vi "Parse Response.vi"(8 "error in (no error)":errorcluster, 10 "Command":T1, 11 "ESM303 in":refnum<class "ESM303.lvclass">) -> (0 "error out":errorcluster, 3 "ESM303 out":refnum<class "ESM303.lvclass">)   [LabVIEW 2018, in "ESM303.lvlib" / "ESM303.lvclass"]
uses:
  ESM303.lvclass
  builds/Force Test Stand.lvlibp/Custom Controls/Commands.ctl
  ESM303.lvclass/ESM303.ctl
  builds/Force Test Stand.lvlibp/Custom Controls/Crosshead Status.ctl
  builds/Force Test Stand.lvlibp/Custom Controls/Operating Mode.ctl
  builds/Force Test Stand.lvlibp/Custom Controls/Limit Switch Status.ctl
  builds/Force Test Stand.lvlibp/Custom Controls/Travel Units.ctl
  builds/Force Test Stand.lvlibp/Custom Controls/Speed Units.ctl
  builds/Force Test Stand.lvlibp/Custom Controls/Force Units.ctl
  builds/Force Test Stand.lvlibp/Force Test Stand.lvclass
  C:/Users/Ron.Dexter.LUMINARTECH/Desktop/builds/Force Test Stand.lvlibp/Force Test Stand.lvclass
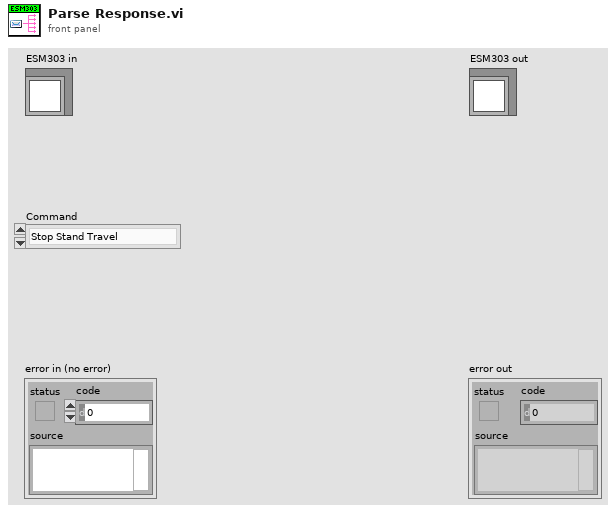
[diagram p1: front panel]
types:
  T1 = typedef "Force Test Stand.lvlibp/Force Test Stand.lvclass/Commands.ctl" = enum16{"Stop Stand Travel", "Start Travel Down (Left)", "Start Travel Up (Right)", "Get Travel Upper Limit", "Get Travel Lower Limit", "Set Travel Upper Limit", "Set Travel Lower Limit", "Get Travel Value", "Set Travel Units (mm)", "Set Travel Units (in)", "Reset Travel to Zero", "Get Speed ", "Set Speed", "Set Speed to Min", "Set Speed to Max", "Get Force Value", "Get Force Units", "Set Force Units (lbF)", "Get Stand Status", "Set Cycle Mode", "Set Limit Mode", "Set Manual Mode", "Set No. Cycles", "Get Travel/Force Values", "Get Completed Cycles", "Get Cycles Setpoint", "Reset Cycles Counter", "Zero Force Gauge", "Set Force Upper Limit", "Set Force Lower Limit", "Get Travel Units", "Get Speed Units", "Default", "Set Force Units (N)", "Set Force Units (kgF)", "Set Force Units (ozF)", "Set Force Units (gF)", "Set Force Real Time Mode", "Set Force Peak Tension Mode", "Set Force Peak Compression Mode", "Set Force High Set-Point", "Set Force Low Set-Point", "Gauge Transmit with Units", "Gauge Transmit w/o Units", "Get Peak Compression Force", "Get Peak Tension Force", "Get Real Time Force", "Disable Force High Limit", "Disable Force Low Limit", "Send Speed Setting to Stand"}
  T2 = typedef "Force Test Stand.lvlibp/Force Test Stand.lvclass/Limit Switch Status.ctl" = enum16{"At Upper Limit", "At Lower Limit", "At No Limit"}
  T3 = typedef "Force Test Stand.lvlibp/Force Test Stand.lvclass/Crosshead Status.ctl" = enum16{"Moving Up (Right)", "Moving Down (Left)", "Stopped"}
  T4 = typedef "Force Test Stand.lvlibp/Force Test Stand.lvclass/Operating Mode.ctl" = enum16{"Cycle", "Limit", "Manual"}
  T5 = typedef "Force Test Stand.lvlibp/Force Test Stand.lvclass/Travel Units.ctl" = enum16{"in", "mm"}
  T6 = typedef "Force Test Stand.lvlibp/Force Test Stand.lvclass/Speed Units.ctl" = enum16{"in/min", "mm/min"}
  T7 = typedef "Force Test Stand.lvlibp/Force Test Stand.lvclass/Force Units.ctl" = enum16{"lbF", "ozF", "gF", "kgF", "N", "kN", "mN"}
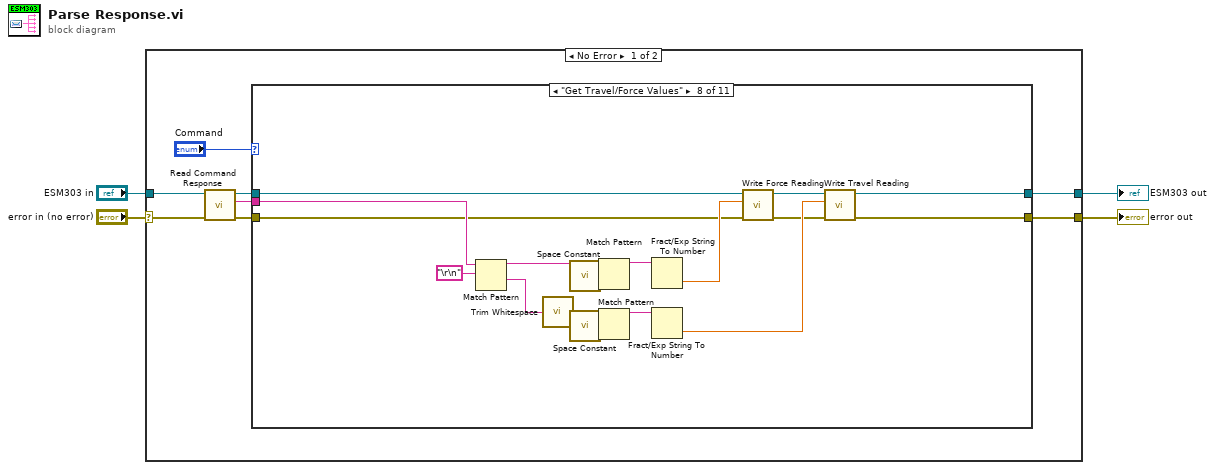
[diagram p0: block diagram]
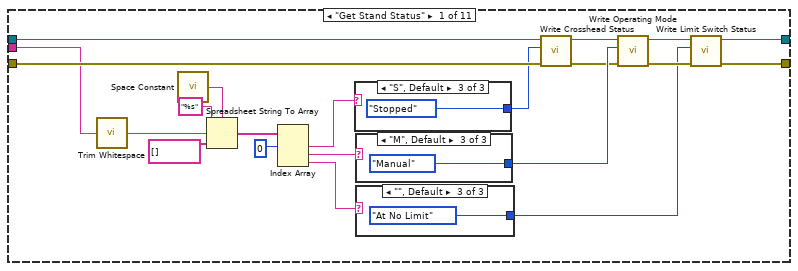
[diagram p2: hidden frame]
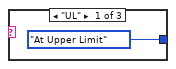
[diagram p3: hidden frame]
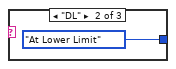
[diagram p4: hidden frame]
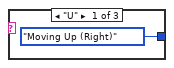
[diagram p5: hidden frame]
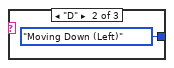
[diagram p6: hidden frame]
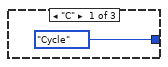
[diagram p7: hidden frame]
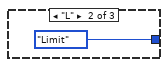
[diagram p8: hidden frame]
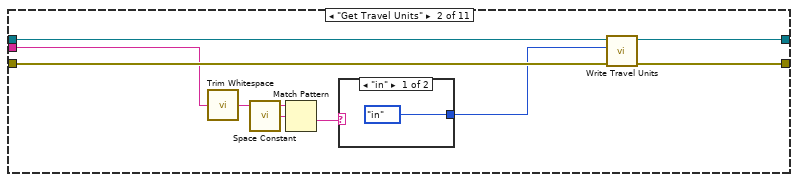
[diagram p9: hidden frame]
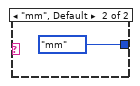
[diagram p10: hidden frame]
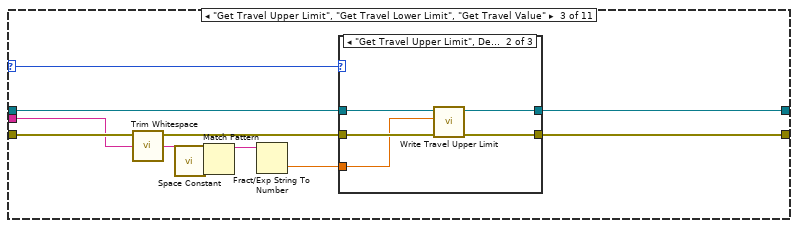
[diagram p11: hidden frame]
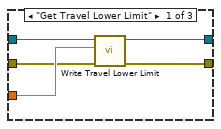
[diagram p12: hidden frame]
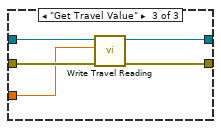
[diagram p13: hidden frame]
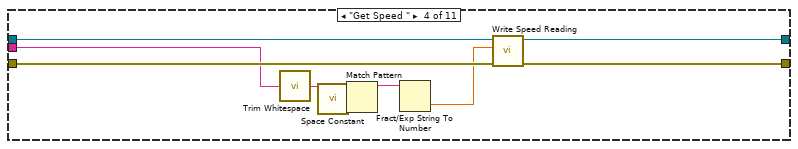
[diagram p14: hidden frame]
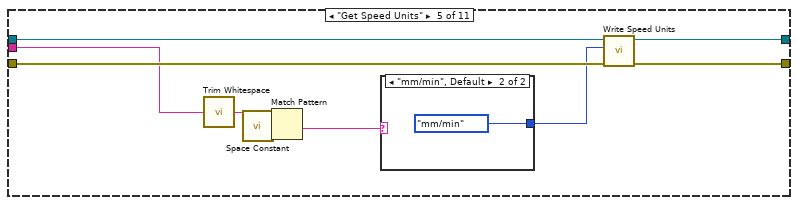
[diagram p15: hidden frame]
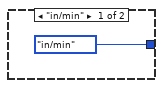
[diagram p16: hidden frame]
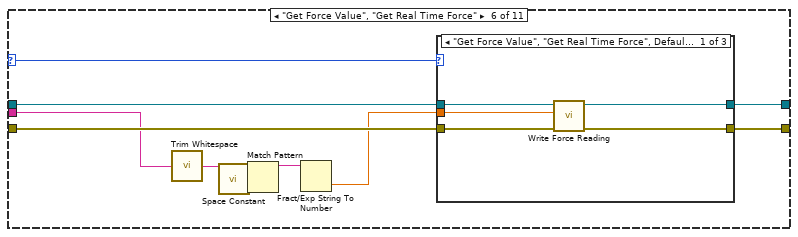
[diagram p17: hidden frame]
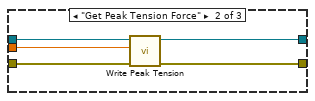
[diagram p18: hidden frame]
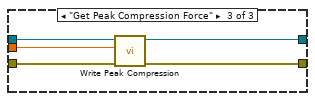
[diagram p19: hidden frame]
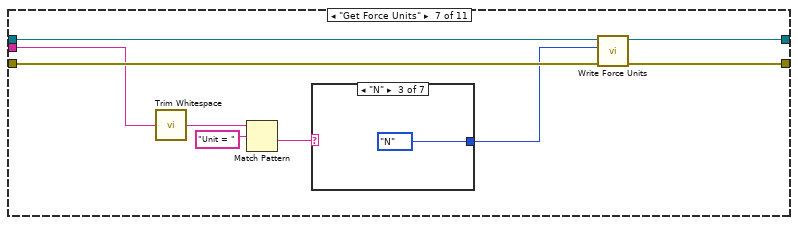
[diagram p20: hidden frame]
diagram:
  n1 = case shown="No Error" "error in (no error)" {
    selector: "error in (no error)" -> [w12 w176]
    tunnel: [w5 w176] -> w3
    tunnel: [w8 w175] -> w1
    tunnel: "ESM303 in" -> [w11 w175]
    frame No Error {
      n2 = call "Read Command Response.vi"("error in (no error)"=w12, "ESM303 in"=w11) -> ("error out"=w6:errorcluster, "Command Response"=w7:string, "ESM303 out"=w10:refnum<class "ESM303.lvclass">)  [unwired: 7 in]
      n3 = case shown="\"Get Travel/Force Values\"" "Command" {
        selector: "Command" -> [_ _ w63 _ _ w99 _ _ _ _ _]
        tunnel: w10 -> [w26 w49 w62 w83 w95 w108 w132 w149 w165 w171 w174]
        tunnel: [w18 w47 w57 w87 w94 w107 w130 w144 w163 w169 w174] -> w8
        tunnel: w7 -> [w14 w44 w55 w80 w89 w101 w125 w156 w160 w167 _]
        tunnel: w6 -> [w25 w48 w61 w82 w92 w106 w131 w146 w164 w170 w173]
        tunnel: [w17 w46 w56 w86 w93 w105 w129 w143 w162 w168 w173] -> w5
        frame "Get Stand Status" {
          n4 = call <vilib>:"Trim Whitespace.vi"("string"=w14) -> ("trimmed string"=w13:string)  [unwired: 1 in]
          n5 = call <vilib>:"Space Constant.vi"() -> ("String"=w15:string)
          n6 = Spreadsheet String To Array(delimiter (Tab)=w15, format string="%s", spreadsheet string=w13, array type (2D Dbl)=string[] []) -> (array=w31:string[])
          n7 = Index Array(array=w31, index #1=0) -> (element #1=w27:string, element #2=w29:string, element #3=w21:string)  [unwired: 2 in]
          n8 = case shown="\"S\", Default" w27 {
            tunnel: [Crosshead_Status."Moving Up (Right)" ("Crosshead Status") Crosshead_Status."Moving Down (Left)" ("Crosshead Status") Crosshead_Status."Stopped" ("Crosshead Status")] -> w22
            frame "U" {
            }
            frame "D" {
            }
            frame "S", Default {
            }
          }
          n9 = case shown="\"M\", Default" w29 {
            tunnel: [Operating_Mode."Cycle" ("Operating Mode") Operating_Mode."Limit" ("Operating Mode") Operating_Mode."Manual" ("Operating Mode")] -> w28
            frame "C" {
            }
            frame "L" {
            }
            frame "M", Default {
            }
          }
          n10 = case shown="\"\", Default" w21 {
            tunnel: [Limit_Switch_Status."At Upper Limit" ("Limit Switch Status") Limit_Switch_Status."At Lower Limit" ("Limit Switch Status") Limit_Switch_Status."At No Limit" ("Limit Switch Status")] -> w16
            frame "UL" {
            }
            frame "DL" {
            }
            frame "", Default {
            }
          }
          n11 = call "Write Crosshead Status.vi"("error in (no error)"=w25, "Crosshead Status"=w22, "Force Test Stand in"=w26) -> ("error out"=w23:errorcluster, "Force Test Stand out"=w24:refnum<class "ESM303.lvclass">)  [unwired: 7 in]
          n12 = call "Write Operating Mode.vi"("error in (no error)"=w23, "Operating Mode"=w28, "Force Test Stand in"=w24) -> ("error out"=w19:errorcluster, "Force Test Stand out"=w20:refnum<class "ESM303.lvclass">)  [unwired: 7 in]
          n13 = call "Write Limit Switch Status.vi"("error in (no error)"=w19, "Limit Switch Status"=w16, "Force Test Stand in"=w20) -> ("error out"=w17:errorcluster, "Force Test Stand out"=w18:refnum<class "ESM303.lvclass">)  [unwired: 7 in]
        }
        frame "Get Travel Units" {
          n14 = call <vilib>:"Trim Whitespace.vi"("string"=w44) -> ("trimmed string"=w43:string)  [unwired: 1 in]
          n15 = call <vilib>:"Space Constant.vi"() -> ("String"=w51:string)
          n16 = Match Pattern(string=w43, regular expression=w51) -> (after substring=w50:string)  [unwired: 1 in, 3 out]
          n17 = case shown="\"in\"" w50 {
            tunnel: [Travel_Units."in" ("Travel Units") Travel_Units."mm" ("Travel Units")] -> w45
            frame "in" {
            }
            frame "mm", Default {
            }
          }
          n18 = call "Write Travel Units.vi"("error in (no error)"=w48, "Travel Units"=w45, "Force Test Stand in"=w49) -> ("error out"=w46:errorcluster, "Force Test Stand out"=w47:refnum<class "ESM303.lvclass">)  [unwired: 7 in]
        }
        frame "Get Travel Upper Limit", "Get Travel Lower Limit", "Get Travel Value" {
          n19 = call <vilib>:"Trim Whitespace.vi"("string"=w55) -> ("trimmed string"=w54:string)  [unwired: 1 in]
          n20 = call <vilib>:"Space Constant.vi"() -> ("String"=w59:string)
          n21 = Match Pattern(string=w54, regular expression=w59) -> (before substring=w58:string)  [unwired: 1 in, 3 out]
          n22 = Fract/Exp String To Number(string=w58) -> (number=w60:dbl)  [unwired: 3 in, 1 out]
          n23 = case shown="\"Get Travel Upper Limit\", Default" w63 {
            tunnel: w62 -> [w68 w73 w76]
            tunnel: [w67 w72 w74] -> w57
            tunnel: w61 -> [w65 w71 w78]
            tunnel: [w64 w70 w77] -> w56
            tunnel: w60 -> [w66 w69 w75]
            frame "Get Travel Lower Limit" {
              n24 = call "Write Travel Lower Limit.vi"("error in (no error)"=w65, "Travel Lower Limit"=w66, "Force Test Stand in"=w68) -> ("error out"=w64:errorcluster, "Force Test Stand out"=w67:refnum<class "ESM303.lvclass">)  [unwired: 7 in]
            }
            frame "Get Travel Upper Limit", Default {
              n25 = call "Write Travel Upper Limit.vi"("error in (no error)"=w71, "Travel Upper Limit"=w69, "Force Test Stand in"=w73) -> ("error out"=w70:errorcluster, "Force Test Stand out"=w72:refnum<class "ESM303.lvclass">)  [unwired: 7 in]
            }
            frame "Get Travel Value" {
              n26 = call "Write Travel Reading.vi"("error in (no error)"=w78, "Travel Reading"=w75, "Force Test Stand in"=w76) -> ("error out"=w77:errorcluster, "Force Test Stand out"=w74:refnum<class "ESM303.lvclass">)  [unwired: 7 in]
            }
          }
        }
        frame "Get Speed " {
          n27 = call <vilib>:"Trim Whitespace.vi"("string"=w80) -> ("trimmed string"=w79:string)  [unwired: 1 in]
          n28 = call <vilib>:"Space Constant.vi"() -> ("String"=w85:string)
          n29 = Match Pattern(string=w79, regular expression=w85) -> (before substring=w84:string)  [unwired: 1 in, 3 out]
          n30 = Fract/Exp String To Number(string=w84) -> (number=w81:dbl)  [unwired: 3 in, 1 out]
          n31 = call "Write Speed Reading.vi"("error in (no error)"=w82, "Speed Reading"=w81, "Force Test Stand in"=w83) -> ("error out"=w86:errorcluster, "Force Test Stand out"=w87:refnum<class "ESM303.lvclass">)  [unwired: 7 in]
        }
        frame "Get Speed Units" {
          n32 = call <vilib>:"Trim Whitespace.vi"("string"=w89) -> ("trimmed string"=w88:string)  [unwired: 1 in]
          n33 = call <vilib>:"Space Constant.vi"() -> ("String"=w96:string)
          n34 = Match Pattern(string=w88, regular expression=w96) -> (after substring=w91:string)  [unwired: 1 in, 3 out]
          n35 = case shown="\"mm/min\", Default" w91 {
            tunnel: [Speed_Units."in/min" ("Speed Units") Speed_Units."mm/min" ("Speed Units")] -> w90
            frame "in/min" {
            }
            frame "mm/min", Default {
            }
          }
          n36 = call "Write Speed Units.vi"("error in (no error)"=w92, "Speed Units"=w90, "Force Test Stand in"=w95) -> ("error out"=w93:errorcluster, "Force Test Stand out"=w94:refnum<class "ESM303.lvclass">)  [unwired: 7 in]
        }
        frame "Get Force Value", "Get Real Time Force" {
          n37 = call <vilib>:"Trim Whitespace.vi"("string"=w101) -> ("trimmed string"=w100:string)  [unwired: 1 in]
          n38 = call <vilib>:"Space Constant.vi"() -> ("String"=w104:string)
          n39 = Match Pattern(string=w100, regular expression=w104) -> (before substring=w103:string)  [unwired: 1 in, 3 out]
          n40 = Fract/Exp String To Number(string=w103) -> (number=w102:dbl)  [unwired: 3 in, 1 out]
          n41 = case shown="\"Get Force Value\", \"Get Real Time Force\", Default" w99 {
            tunnel: w108 -> [w113 w115 w122]
            tunnel: [w112 w116 w120] -> w107
            tunnel: w106 -> [w111 w118 w123]
            tunnel: [w110 w117 w119] -> w105
            tunnel: w102 -> [w109 w114 w121]
            frame "Get Force Value", "Get Real Time Force", Default {
              n42 = call "Write Force Reading.vi"("error in (no error)"=w111, "Force Reading"=w109, "Force Test Stand in"=w113) -> ("error out"=w110:errorcluster, "Force Test Stand out"=w112:refnum<class "ESM303.lvclass">)  [unwired: 7 in]
            }
            frame "Get Peak Tension Force" {
              n43 = call "Write Peak Tension.vi"("error in (no error)"=w118, "Peak Tension"=w114, "Force Test Stand in"=w115) -> ("error out"=w117:errorcluster, "Force Test Stand out"=w116:refnum<class "ESM303.lvclass">)  [unwired: 7 in]
            }
            frame "Get Peak Compression Force" {
              n44 = call "Write Peak Compression.vi"("error in (no error)"=w123, "Peak Compression"=w121, "Force Test Stand in"=w122) -> ("error out"=w119:errorcluster, "Force Test Stand out"=w120:refnum<class "ESM303.lvclass">)  [unwired: 7 in]
            }
          }
        }
        frame "Get Force Units" {
          n45 = call <vilib>:"Trim Whitespace.vi"("string"=w125) -> ("trimmed string"=w124:string)  [unwired: 1 in]
          n46 = Match Pattern(string=w124, regular expression="Unit = ") -> (after substring=w127:string)  [unwired: 1 in, 3 out]
          n47 = case shown="\"N\"" w127 {
            tunnel: [Force_Units."lbF" ("Force Units") Force_Units."ozF" ("Force Units") Force_Units."N" ("Force Units") Force_Units."gF" ("Force Units") Force_Units."kgF" ("Force Units") Force_Units."kN" ("Force Units") Force_Units."mN" ("Force Units")] -> w128
            frame "lb" {
            }
            frame "oz" {
            }
            frame "N" {
            }
            frame "g" {
            }
            frame "kg" {
            }
            frame "kN" {
            }
            frame "mN", Default {
            }
          }
          n48 = call "Write Force Units.vi"("error in (no error)"=w131, "Force Units"=w128, "Force Test Stand in"=w132) -> ("error out"=w129:errorcluster, "Force Test Stand out"=w130:refnum<class "ESM303.lvclass">)  [unwired: 7 in]
        }
        frame "Get Travel/Force Values" {
          n49 = Match Pattern(string=w156, regular expression="\r\n") -> (before substring=w153:string, after substring=w141:string)  [unwired: 1 in, 2 out]
          n50 = call <vilib>:"Trim Whitespace.vi"("string"=w141) -> ("trimmed string"=w140:string)  [unwired: 1 in]
          n51 = call <vilib>:"Space Constant.vi"() -> ("String"=w155:string)
          n52 = call <vilib>:"Space Constant.vi"() -> ("String"=w152:string)
          n53 = Match Pattern(string=w153, regular expression=w155) -> (before substring=w154:string)  [unwired: 1 in, 3 out]
          n54 = Match Pattern(string=w140, regular expression=w152) -> (before substring=w151:string)  [unwired: 1 in, 3 out]
          n55 = Fract/Exp String To Number(string=w154) -> (number=w147:dbl)  [unwired: 3 in, 1 out]
          n56 = Fract/Exp String To Number(string=w151) -> (number=w150:dbl)  [unwired: 3 in, 1 out]
          n57 = call "Write Force Reading.vi"("error in (no error)"=w146, "Force Reading"=w147, "Force Test Stand in"=w149) -> ("error out"=w145:errorcluster, "Force Test Stand out"=w148:refnum<class "ESM303.lvclass">)  [unwired: 7 in]
          n58 = call "Write Travel Reading.vi"("error in (no error)"=w145, "Travel Reading"=w150, "Force Test Stand in"=w148) -> ("error out"=w143:errorcluster, "Force Test Stand out"=w144:refnum<class "ESM303.lvclass">)  [unwired: 7 in]
        }
        frame "Get Completed Cycles" {
          n59 = call <vilib>:"Trim Whitespace.vi"("string"=w160) -> ("trimmed string"=w159:string)  [unwired: 1 in]
          n60 = Match Pattern(string=w159, regular expression=" Cycles") -> (before substring=w157:string)  [unwired: 1 in, 3 out]
          n61 = Fract/Exp String To Number(string=w157) -> (number=w161:dbl)  [unwired: 3 in, 1 out]
          n62 = call "Write Cycles Completed.vi"("error in (no error)"=w164, "Cycles Completed"=w161, "Force Test Stand in"=w165) -> ("error out"=w162:errorcluster, "Force Test Stand out"=w163:refnum<class "ESM303.lvclass">)  [unwired: 7 in]
        }
        frame "Get Cycles Setpoint" {
          n63 = call <vilib>:"Trim Whitespace.vi"("string"=w167) -> ("trimmed string"=w166:string)  [unwired: 1 in]
          n64 = Fract/Exp String To Number(string=w166) -> (number=w172:dbl)  [unwired: 3 in, 1 out]
          n65 = call "Write Cycles Setpoint.vi"("error in (no error)"=w170, "Cycles Setpoint"=w172, "Force Test Stand in"=w171) -> ("error out"=w168:errorcluster, "Force Test Stand out"=w169:refnum<class "ESM303.lvclass">)  [unwired: 7 in]
        }
        frame Default {
        }
      }
    }
    frame Error {
    }
  }
  "error out" <- w3
  "ESM303 out" <- w1
